vi "LIA-SR865A.vi"(0 "VISA resource name":refnum<visa-resource-name>="LIA", 1 "SubVI":bool, 5 "Input cluster":T1, 11 "error in (no error)":errorcluster) -> (4 "VISA resource name out":refnum<visa-resource-name>, 6 "output cluster":T1, 15 "error out":errorcluster)   [LabVIEW 2016]
uses:
  <instrlib>/Stanford Research SR865/Stanford Research SR865.lvlib
panel:
  out "On":bool
  out "On":bool
  in  "?":bool
  in  "?":bool
  out "On":bool
  out "On":bool
  in  "?":bool
  in  "?":bool
  in  "?":bool
  out "On":bool
  in  "?":bool
  out "On":bool
  in  "CH2 Offset":dbl min=-999.99 max=999.99 format="%#.2f"
  in  "CH1 Offset":dbl min=-999.99 max=999.99 format="%#.2f"
  in  "?":i32=1 min=1 max=99 step=1
  in  "?":bool
  out "On":bool
  in  "Trig":string(combo)="0"
  in  "?":bool
  out "On":bool
  in  "Slope":string(combo)="3"
  in  "Range":enum32{"1 mA", "10 nA"}(radio)
  in  "0":string(combo)="0"
  in  "Input":enum32{"50 W", "1 MW"}(radio)=enum."1 MW"
  in  "?":bool
  in  "Input Shields":enum32{"Float", "Ground"}(radio)=enum."Ground"
  in  "Couple":enum32{"AC", "DC"}(radio)
  in  "A-B":enum32{"A", "A-B"}(radio)
  in  "Mode":enum32{"Common", "Difference"}(radio)
  in  "Input":enum32{"Voltage", "Current"}(radio)
  in  "?":bool
  in  "DC Level":dbl min=-5.0 max=5.0 format="%.3f"
  in  "?":bool
  in  "Input Range":string(combo)="1"
  in  "?":bool
  in  "Amplitude":dbl=2.0 min=1e-09 max=2.0 format="%.3g"
  in  "Internal Ref\nFrequency":dbl=25.0 min=0.0 format="%.4f"
  in  "?":ext=-1.9354838709677438 format="%#.3g"
  in  "Expand":string(combo)="0"
  in  "CH2 Output":string(combo)="1"
  in  "Expand":string(combo)="0"
  in  "CH1 Output":string(combo)="1"
  in  "1":string(combo)="1"
  in  "Time Constant":string(combo)="0"
  in  "1":string(combo)="1"
  in  "Sensitivity":string(combo)="0"
  # "Signal"
  # "Reference"
  # "Sine Out"
  # "Phase"
  # "V"
  # "V"
  # "mV"
  # "External"
  # "Ref Source"
  # "kHz"
  # "Current"
  # "Voltage"
  # "Harmonic"
  # "Output"
  # "%"
  # "%"
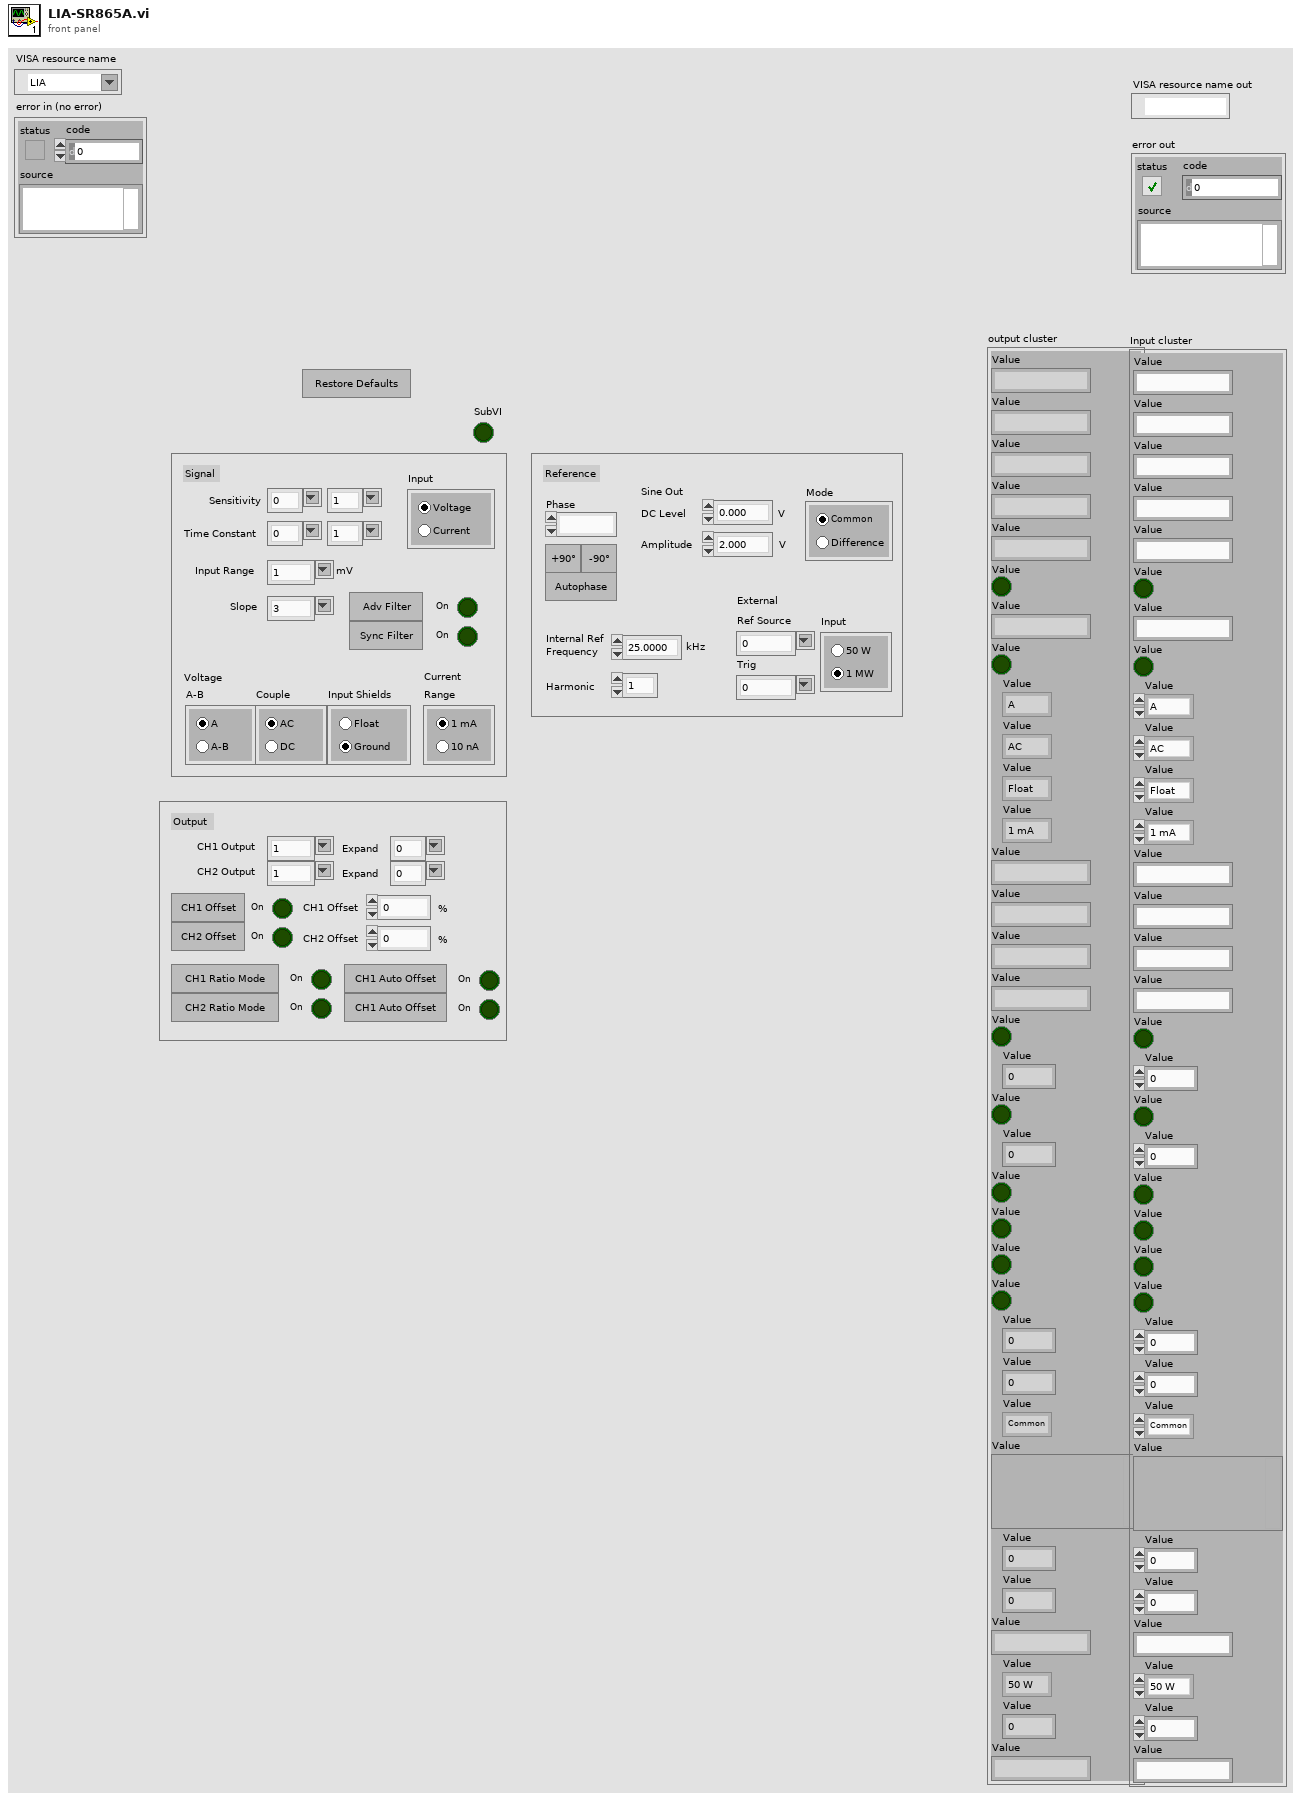
[diagram p1: front panel]
types:
  T1 = cluster{"Value":string, "Value":string, "Value":string, "Value":string, "Value":string, "Value":bool, "Value":string, "Value":bool, "Value":enum32{"A", "A-B"}, "Value":enum32{"AC", "DC"}, "Value":enum32{"Float", "Ground"}, "Value":enum32{"1 mA", "10 nA"}, "Value":string, "Value":string, "Value":string, "Value":string, "Value":bool, "Value":dbl, "Value":bool, "Value":dbl, "Value":bool, "Value":bool, "Value":bool, "Value":bool, "Value":ext, "Value":dbl, "Value":enum32{"Common", "Difference"}, "Value":variant, "Value":dbl, "Value":dbl, "Value":string, "Value":enum32{"50 W", "1 MW"}, "Value":i32, "Value":string}
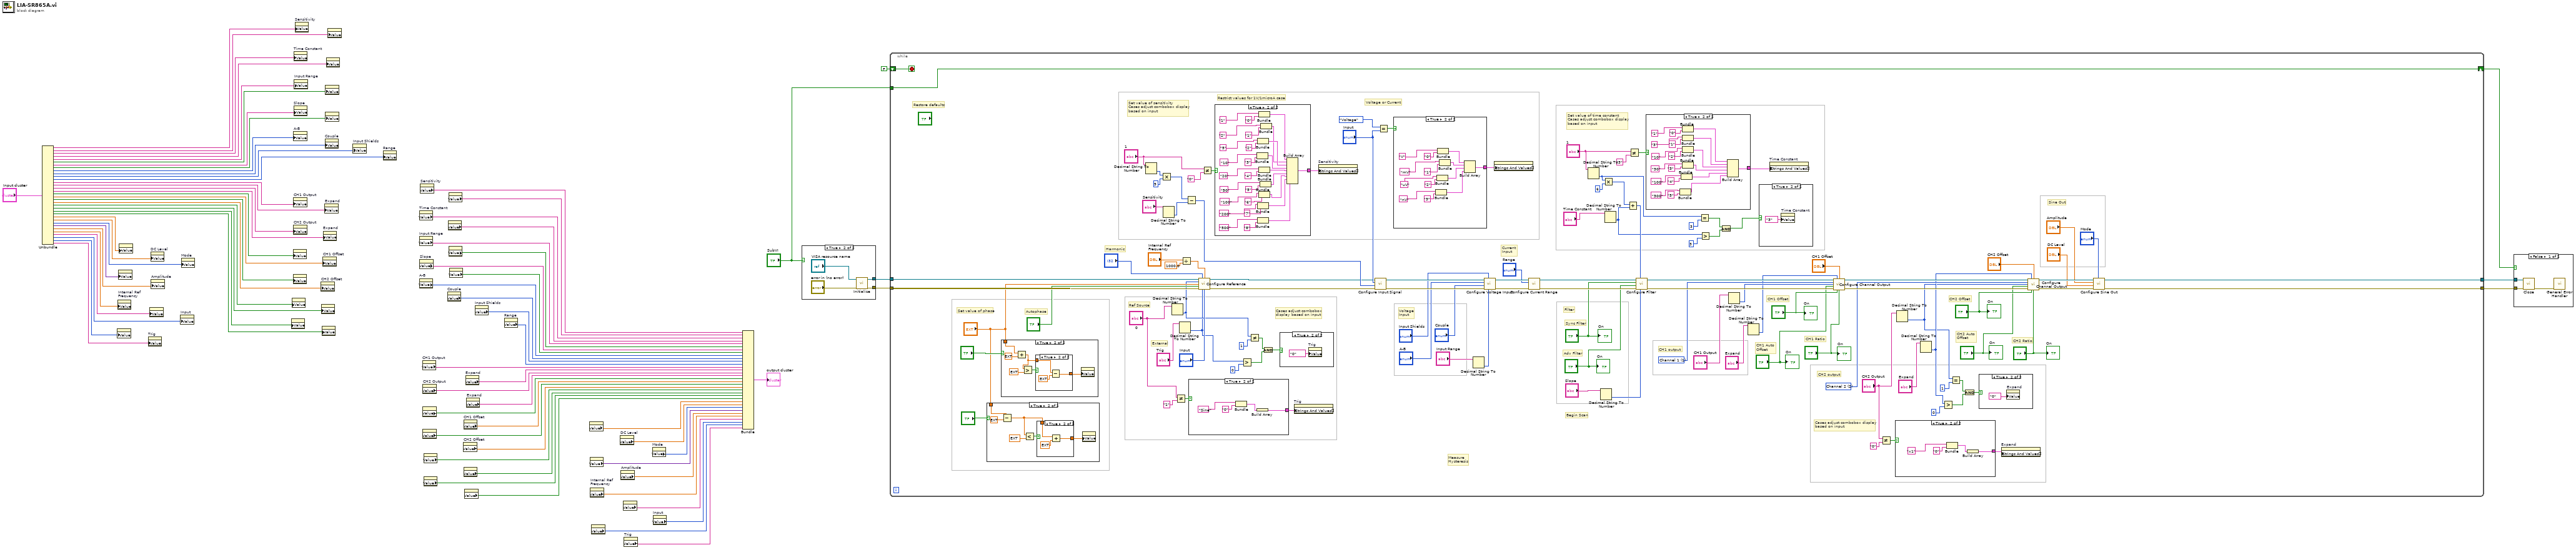
[diagram p0: block diagram]
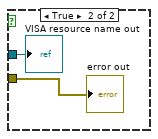
[diagram p2: hidden frame]
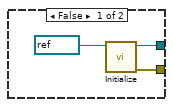
[diagram p3: hidden frame]
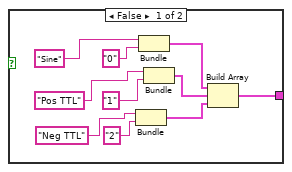
[diagram p4: hidden frame]
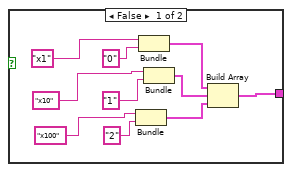
[diagram p7: hidden frame]
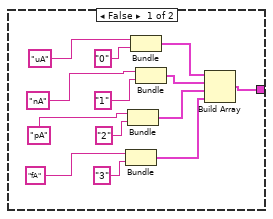
[diagram p9: hidden frame]
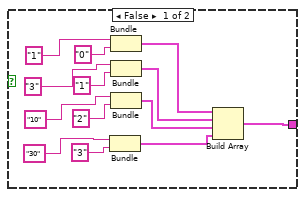
[diagram p14: hidden frame]
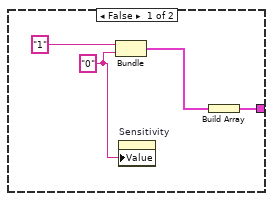
[diagram p15: hidden frame]
diagram:
  n1 = Unbundle("Input cluster") -> ("Value"=w42:string, "Value"=w41:string, "Value"=w40:string, "Value"=w39:string, "Value"=w38:string, "Value"=w37:bool, "Value"=w36:string, "Value"=w35:bool, "Value"=w34:enum32{"A", "A-B"}, "Value"=w33:enum32{"AC", "DC"}, "Value"=w32:enum32{"Float", "Ground"}, "Value"=w31:enum32{"1 mA", "10 nA"}, "Value"=w30:string, "Value"=w29:string, "Value"=w28:string, "Value"=w27:string, "Value"=w26:bool, "Value"=w25:dbl, "Value"=w24:bool, "Value"=w23:dbl, "Value"=w22:bool, "Value"=w21:bool, "Value"=w20:bool, "Value"=w19:bool, "Value"=w18:ext, "Value"=w17:dbl, "Value"=w16:enum32{"Common", "Difference"}, "Value"=w15:variant, "Value"=w14:dbl, "Value"=w13:dbl, "Value"=w12:string, "Value"=w11:enum32{"50 W", "1 MW"}, "Value"=w10:i32, "Value"=w9:string)
  n2 = property class="DigNum (strict)"("Value"=w10) -> ()  [unwired: 2 in, 2 out]
  n3 = property on="Internal Ref\nFrequency" class="DigNum (strict)"("Value"=w13) -> ()  [unwired: 2 in, 2 out]
  n4 = property class="Bool"("Value"=w15) -> ()  [unwired: 2 in, 2 out]
  n5 = property class="DigNum (strict)"("Value"=w18) -> ()  [unwired: 2 in, 2 out]
  n6 = property on="Trig" class="CmbBox"("Value"=w9) -> ()  [unwired: 2 in, 2 out]
  n7 = property class="CmbBox"("Value"=w12) -> ()  [unwired: 2 in, 2 out]
  n8 = property on="DC Level" class="DigNum (strict)"("Value"=w17) -> ()  [unwired: 2 in, 2 out]
  n9 = property on="Amplitude" class="DigNum (strict)"("Value"=w14) -> ()  [unwired: 2 in, 2 out]
  n10 = property on="Input" class="RadioBtnsControl (strict)"("Value"=w11) -> ()  [unwired: 2 in, 2 out]
  n11 = property on="Mode" class="RadioBtnsControl (strict)"("Value"=w16) -> ()  [unwired: 2 in, 2 out]
  n12 = property class="Bool (strict)"("Value"=w20) -> ()  [unwired: 2 in, 2 out]
  n13 = property class="Bool (strict)"("Value"=w22) -> ()  [unwired: 2 in, 2 out]
  n14 = property class="Bool (strict)"("Value"=w26) -> ()  [unwired: 2 in, 2 out]
  n15 = property class="Bool (strict)"("Value"=w24) -> ()  [unwired: 2 in, 2 out]
  n16 = property on="A-B" class="RadioBtnsControl (strict)"("Value"=w34) -> ()  [unwired: 2 in, 2 out]
  n17 = property on="CH1 Output" class="CmbBox"("Value"=w30) -> ()  [unwired: 2 in, 2 out]
  n18 = property on="CH2 Output" class="CmbBox"("Value"=w28) -> ()  [unwired: 2 in, 2 out]
  n19 = property on="Time Constant" class="CmbBox"("Value"=w40) -> ()  [unwired: 2 in, 2 out]
  n20 = property on="Slope" class="CmbBox"("Value"=w36) -> ()  [unwired: 2 in, 2 out]
  n21 = property on="Input Range" class="CmbBox"("Value"=w38) -> ()  [unwired: 2 in, 2 out]
  n22 = property on="Sensitivity" class="CmbBox"("Value"=w42) -> ()  [unwired: 2 in, 2 out]
  n23 = property on="CH2 Offset" class="DigNum (strict)"("Value"=w23) -> ()  [unwired: 2 in, 2 out]
  n24 = property class="Bool (strict)"("Value"=w21) -> ()  [unwired: 2 in, 2 out]
  n25 = property class="Bool (strict)"("Value"=w19) -> ()  [unwired: 2 in, 2 out]
  n26 = property on="CH1 Offset" class="DigNum (strict)"("Value"=w25) -> ()  [unwired: 2 in, 2 out]
  n27 = property on="Expand" class="CmbBox"("Value"=w27) -> ()  [unwired: 2 in, 2 out]
  n28 = property on="Expand" class="CmbBox"("Value"=w29) -> ()  [unwired: 2 in, 2 out]
  n29 = property on="Couple" class="RadioBtnsControl (strict)"("Value"=w33) -> ()  [unwired: 2 in, 2 out]
  n30 = property class="Bool (strict)"("Value"=w37) -> ()  [unwired: 2 in, 2 out]
  n31 = property class="Bool (strict)"("Value"=w35) -> ()  [unwired: 2 in, 2 out]
  n32 = property class="CmbBox"("Value"=w39) -> ()  [unwired: 2 in, 2 out]
  n33 = property class="CmbBox"("Value"=w41) -> ()  [unwired: 2 in, 2 out]
  n34 = property on="Input Shields" class="RadioBtnsControl (strict)"("Value"=w32) -> ()  [unwired: 2 in, 2 out]
  n35 = property on="Range" class="RadioBtnsControl (strict)"("Value"=w31) -> ()  [unwired: 2 in, 2 out]
  n36 = property on="Time Constant" class="CmbBox"() -> ("Value"=w74:string)  [unwired: 2 in, 2 out]
  n37 = property on="Input Range" class="CmbBox"() -> ("Value"=w72:string)  [unwired: 2 in, 2 out]
  n38 = property on="A-B" class="RadioBtnsControl (strict)"() -> ("Value"=w68:enum32{"A", "A-B"})  [unwired: 2 in, 2 out]
  n39 = property on="Slope" class="CmbBox"() -> ("Value"=w70:string)  [unwired: 2 in, 2 out]
  n40 = property on="Sensitivity" class="CmbBox"() -> ("Value"=w76:string)  [unwired: 2 in, 2 out]
  n41 = property on="CH1 Output" class="CmbBox"() -> ("Value"=w64:string)  [unwired: 2 in, 2 out]
  n42 = property on="CH2 Output" class="CmbBox"() -> ("Value"=w62:string)  [unwired: 2 in, 2 out]
  n43 = property class="Bool (strict)"() -> ("Value"=w60:bool)  [unwired: 2 in, 2 out]
  n44 = property class="Bool (strict)"() -> ("Value"=w58:bool)  [unwired: 2 in, 2 out]
  n45 = property class="Bool (strict)"() -> ("Value"=w56:bool)  [unwired: 2 in, 2 out]
  n46 = property class="Bool (strict)"() -> ("Value"=w54:bool)  [unwired: 2 in, 2 out]
  n47 = property on="Couple" class="RadioBtnsControl (strict)"() -> ("Value"=w67:enum32{"AC", "DC"})  [unwired: 2 in, 2 out]
  n48 = property class="CmbBox"() -> ("Value"=w73:string)  [unwired: 2 in, 2 out]
  n49 = property class="CmbBox"() -> ("Value"=w75:string)  [unwired: 2 in, 2 out]
  n50 = property class="Bool (strict)"() -> ("Value"=w71:bool)  [unwired: 2 in, 2 out]
  n51 = property class="Bool (strict)"() -> ("Value"=w69:bool)  [unwired: 2 in, 2 out]
  n52 = property on="CH2 Offset" class="DigNum (strict)"() -> ("Value"=w57:dbl)  [unwired: 2 in, 2 out]
  n53 = property on="CH1 Offset" class="DigNum (strict)"() -> ("Value"=w59:dbl)  [unwired: 2 in, 2 out]
  n54 = property class="Bool (strict)"() -> ("Value"=w55:bool)  [unwired: 2 in, 2 out]
  n55 = property class="Bool (strict)"() -> ("Value"=w53:bool)  [unwired: 2 in, 2 out]
  n56 = property on="Expand" class="CmbBox"() -> ("Value"=w63:string)  [unwired: 2 in, 2 out]
  n57 = property on="Expand" class="CmbBox"() -> ("Value"=w61:string)  [unwired: 2 in, 2 out]
  n58 = property on="Input Shields" class="RadioBtnsControl (strict)"() -> ("Value"=w66:enum32{"Float", "Ground"})  [unwired: 2 in, 2 out]
  n59 = property on="Range" class="RadioBtnsControl (strict)"() -> ("Value"=w65:enum32{"1 mA", "10 nA"})  [unwired: 2 in, 2 out]
  n60 = property class="DigNum (strict)"() -> ("Value"=w52:ext)  [unwired: 2 in, 2 out]
  n61 = property class="Bool"() -> ("Value"=w49:variant)  [unwired: 2 in, 2 out]
  n62 = property on="Internal Ref\nFrequency" class="DigNum (strict)"() -> ("Value"=w47:dbl)  [unwired: 2 in, 2 out]
  n63 = property class="DigNum (strict)"() -> ("Value"=w44:i32)  [unwired: 2 in, 2 out]
  n64 = property on="DC Level" class="DigNum (strict)"() -> ("Value"=w51:dbl)  [unwired: 2 in, 2 out]
  n65 = property on="Amplitude" class="DigNum (strict)"() -> ("Value"=w48:dbl)  [unwired: 2 in, 2 out]
  n66 = property class="CmbBox"() -> ("Value"=w46:string)  [unwired: 2 in, 2 out]
  n67 = property on="Trig" class="CmbBox"() -> ("Value"=w43:string)  [unwired: 2 in, 2 out]
  n68 = property on="Mode" class="RadioBtnsControl (strict)"() -> ("Value"=w50:enum32{"Common", "Difference"})  [unwired: 2 in, 2 out]
  n69 = property on="Input" class="RadioBtnsControl (strict)"() -> ("Value"=w45:enum32{"50 W", "1 MW"})  [unwired: 2 in, 2 out]
  n70 = Bundle("Value"=w76, "Value"=w75, "Value"=w74, "Value"=w73, "Value"=w72, "Value"=w71, "Value"=w70, "Value"=w69, "Value"=w68, "Value"=w67, "Value"=w66, "Value"=w65, "Value"=w64, "Value"=w63, "Value"=w62, "Value"=w61, "Value"=w60, "Value"=w59, "Value"=w58, "Value"=w57, "Value"=w56, "Value"=w55, "Value"=w54, "Value"=w53, "Value"=w52, "Value"=w51, "Value"=w50, "Value"=w49, "Value"=w48, "Value"=w47, "Value"=w46, "Value"=w45, "Value"=w44, "Value"=w43) -> (→"output cluster":T1)  [unwired: 1 in]
  n71 = case shown="True" "SubVI" {
    tunnel: [w79 w84] -> w6
    tunnel: [w78 w83] -> w5
    frame False {
      n72 = call <instrlib>:"Initialize.vi"("VISA resource name"=refnum<visa-resource-name> "LIA") -> ("error out"=w78:errorcluster, "VISA resource name out"=w79:refnum<visa-resource-name>)  [unwired: 9 in]
    }
    frame True {
      n73 = call <instrlib>:"Initialize.vi"("error in (no error)"="error in (no error)", "VISA resource name"="VISA resource name") -> ("error out"=w83:errorcluster, "VISA resource name out"=w84:refnum<visa-resource-name>)  [unwired: 8 in]
    }
  }
  n74 = while {
    tunnel: w6 -> [w180]
    tunnel: w5 -> [w179]
    tunnel: [w87] -> w4
    tunnel: [w86] -> w3
    shift-right: [w85] -> w2
    shift-left: FALSE ("SubVI") -> [w93]
    tunnel: "SubVI" -> [w85]
    stop <- w93 stop-if-true
    w132 = 2 items=["Channel 1"=1, "Channel 2"=2] ("Channel Name (1: Channel 1)")
    w133 = 1 items=["Channel 1"=1, "Channel 2"=2] ("Channel Name (1: Channel 1)")
    # "CH2 Auto\nOffset"
    # "CH1 Auto\nOffset"
    # "CH1 Ratio"
    # "CH2 Ratio"
    # "CH2 Offset"
    # "CH1 Offset"
    # "Sine Out"
    # "Cases adjust combobox\ndisplay based on input"
    # "Cases adjust combobox display\nbased on input"
    # "CH2 output"
    # "Filter"
    # "Current\nInput"
    # "Sync Filter"
    # "Restrict values for 1V/1microA case"
    # "Voltage or Current"
    # "Autophase"
    # "Harmonic"
    # "Begin Scan"
    # "Measure\nHysteresis"
    # "Ref Source"
    # "External"
    # "Adv Filter"
    # "Restore defaults"
    # "Voltage\nInput"
    # "Set value of phase"
    # "CH1 output"
    # "Set value of time constant\nCases adjust combobox display\nbased on input"
    # "Set value of sensitivity\nCases adjust combobox display\nbased on input"
    n75 = case shown="True" "?" {
      tunnel: "?" -> [_ w266]
      frame False {
      }
      frame True {
        n76 = Subtract(x=w266, y=ext 90.0) -> (x-y=w262:ext)
        n77 = Less?(x=w262, y=ext -180.0) -> (x < y?=w263:bool)
        n78 = case shown="True" w263 {
          tunnel: w262 -> [w267 w269]
          tunnel: [w267 w268] -> w261
          frame False {
          }
          frame True {
            n79 = Add(x=w269, y=ext 360.0) -> (x+y=w268:ext)
          }
        }
        n80 = property class="DigNum (strict)"("Value"=w261) -> ()  [unwired: 2 in, 2 out]
      }
    }
    n81 = case shown="True" "?" {
      tunnel: "?" -> [_ w256]
      frame False {
      }
      frame True {
        n82 = Add(x=w256, y=ext 90.0) -> (x+y=w252:ext)
        n83 = Greater?(x=w252, y=ext 180.0) -> (0:w254:bool)
        n84 = case shown="True" w254 {
          tunnel: w252 -> [w257 w260]
          tunnel: [w257 w258] -> w251
          frame False {
          }
          frame True {
            n85 = Subtract(x=w260, y=ext 360.0) -> (x-y=w258:ext)
          }
        }
        n86 = property class="DigNum (strict)"("Value"=w251) -> ()  [unwired: 2 in, 2 out]
      }
    }
    n87 = Decimal String To Number(string="1") -> (number=w176:i32)  [unwired: 2 in, 1 out]
    n88 = Multiply(x=w176, y=9) -> (x*y=w173:i32)
    n89 = Decimal String To Number(string="Sensitivity") -> (number=w174:i32)  [unwired: 2 in, 1 out]
    n90 = Decimal String To Number(string="0") -> (number=w114:i32)  [unwired: 2 in, 1 out]
    n91 = Not Equal?(x="0", y="1") -> (x != y?=w109:bool)
    n92 = Decimal String To Number(string="Trig") -> (number=w112:i32)  [unwired: 2 in, 1 out]
    n93 = Divide(x="Internal Ref\nFrequency", y=1000.0) -> (x/y=w89:dbl)
    n94 = Subtract(x=w173, y=w174) -> (x-y=w149:i32)
    n95 = case shown="True" w109 {
      tunnel: [w197 w204] -> w108
      frame False {
        n96 = Bundle("Neg TTL", "2") -> (w194:cluster{string, string})  [unwired: 1 in]
        n97 = Bundle("Sine", "0") -> (w196:cluster{string, string})  [unwired: 1 in]
        n98 = Bundle("Pos TTL", "1") -> (w195:cluster{string, string})  [unwired: 1 in]
        n99 = Build Array(w196, w195, w194) -> (w197:cluster{string, string}[])
      }
      frame True {
        n100 = Bundle("Sine", "0") -> (w205:cluster{string, string})  [unwired: 1 in]
        n101 = Build Array(w205) -> (w204:cluster{string, string}[])
      }
    }
    n102 = call <instrlib>:"Configure Reference.vi"("VISA resource name"=w180, "Detection Harmonic Number (1)"="?", "Internal Reference Frequency (100000Hz)"=w89, "Reference Source (0: Internal)"=w114, "Manual Phase (0 Degree)"="?", "Auto Phase(0:Disabled)"="?", "error in (no error)"=w179, "External Reference Trigger (0: Sine Zero Crossing)"=w112, "External Reference Trigger Input (0: 50OHMS)"="Input") -> ("VISA resource name out"=w92:refnum<visa-resource-name>, "error out"=w91:errorcluster)  [unwired: 5 in]
    n103 = Not Equal?(x="1", y="0") -> (x != y?=w193:bool)
    n104 = case shown="True" w193 {
      tunnel: [w305 w307] -> w172
      frame False {
        w303 = "0"
        n105 = Bundle("1", w303) -> (w304:cluster{string, string})  [unwired: 1 in]
        n106 = property on="Sensitivity" class="CmbBox"("Value"=w303) -> ()  [unwired: 2 in, 2 out]
        n107 = Build Array(w304) -> (w305:cluster{string, string}[])
      }
      frame True {
        n108 = Bundle("10", "3") -> (w331:cluster{string, string})  [unwired: 1 in]
        n109 = Bundle("5", "2") -> (w333:cluster{string, string})  [unwired: 1 in]
        n110 = Bundle("200", "7") -> (w327:cluster{string, string})  [unwired: 1 in]
        n111 = Bundle("500", "8") -> (w326:cluster{string, string})  [unwired: 1 in]
        n112 = Bundle("1", "0") -> (w334:cluster{string, string})  [unwired: 1 in]
        n113 = Bundle("100", "6") -> (w328:cluster{string, string})  [unwired: 1 in]
        n114 = Bundle("20", "4") -> (w330:cluster{string, string})  [unwired: 1 in]
        n115 = Bundle("50", "5") -> (w329:cluster{string, string})  [unwired: 1 in]
        n116 = Bundle("2", "1") -> (w332:cluster{string, string})  [unwired: 1 in]
        n117 = Build Array(w334, w332, w333, w331, w330, w329, w328, w327, w326) -> (w307:cluster{string, string}[])
      }
    }
    n118 = Greater?(x=w112, y=0) -> (0:w115:bool)
    n119 = Not Equal?(x=w114, y=1) -> (x != y?=w113:bool)
    n120 = And(x=w113, y=w115) -> (x .and. y?=w111:bool)
    n121 = case shown="True" w111 {
      frame False {
      }
      frame True {
        n122 = property on="Trig" class="CmbBox"("Value"="0" ("Trig")) -> ()  [unwired: 2 in, 2 out]
      }
    }
    n123 = property on="Trig" class="CmbBox"("Strings And Values[]"=w108) -> ()  [unwired: 2 in, 2 out]
    n124 = property on="Sensitivity" class="CmbBox"("Strings And Values[]"=w172) -> ()  [unwired: 2 in, 2 out]
    n125 = call <instrlib>:"Configure Input Signal.vi"("error in (no error)"=w91, "Sensitivity (0: 1 V [uA])"=w149, "Signal Input (0: Voltage)"="Input", "VISA resource name"=w92) -> ("error out"=w185:errorcluster, "VISA resource name out"=w181:refnum<visa-resource-name>)  [unwired: 6 in]
    n126 = Equal?(x=enum32{"Voltage", "Current"}."Voltage" ("y"), y="Input") -> (x = y?=w168:bool)
    n127 = case shown="True" w168 {
      tunnel: [w225 w242] -> w167
      frame False {
        n128 = Bundle("fA", "3") -> (w226:cluster{string, string})  [unwired: 1 in]
        n129 = Bundle("pA", "2") -> (w227:cluster{string, string})  [unwired: 1 in]
        n130 = Bundle("uA", "0") -> (w229:cluster{string, string})  [unwired: 1 in]
        n131 = Bundle("nA", "1") -> (w228:cluster{string, string})  [unwired: 1 in]
        n132 = Build Array(w229, w228, w227, w226) -> (w225:cluster{string, string}[])
      }
      frame True {
        n133 = Bundle("nV", "3") -> (w238:cluster{string, string})  [unwired: 1 in]
        n134 = Bundle("uV", "2") -> (w239:cluster{string, string})  [unwired: 1 in]
        n135 = Bundle("V", "0") -> (w241:cluster{string, string})  [unwired: 1 in]
        n136 = Bundle("mV", "1") -> (w240:cluster{string, string})  [unwired: 1 in]
        n137 = Build Array(w241, w240, w239, w238) -> (w242:cluster{string, string}[])
      }
    }
    n138 = Decimal String To Number(string="Input Range") -> (number=w140:i32)  [unwired: 2 in, 1 out]
    n139 = call <instrlib>:"Configure Voltage Input.vi"("Voltage Input Range (0: 1V)"=w140, "Voltage Input Shields (0: Float)"="Input Shields", "error in (no error)"=w185, "Voltage Input Coupling (0: AC)"="Couple", "Voltage Input Mode (0: A)"="A-B", "VISA resource name"=w181) -> ("error out"=w186:errorcluster, "VISA resource name out"=w182:refnum<visa-resource-name>)  [unwired: 4 in]
    n140 = property class="CmbBox"("Strings And Values[]"=w167) -> ()  [unwired: 2 in, 2 out]
    n141 = call <instrlib>:"Configure Current Range.vi"("error in (no error)"=w186, "Current Input Gain (0: 1MOmega(1uA))"="Range", "VISA resource name"=w182) -> ("error out"=w187:errorcluster, "VISA resource name out"=w183:refnum<visa-resource-name>)  [unwired: 7 in]
    n142 = Decimal String To Number(string="1") -> (number=w161:i32)  [unwired: 2 in, 1 out]
    n143 = Decimal String To Number(string="Slope") -> (number=w152:i32)  [unwired: 2 in, 1 out]
    n144 = Multiply(x=w161, y=6) -> (x*y=w165:i32)
    n145 = Decimal String To Number(string="Time Constant") -> (number=w160:i32)  [unwired: 2 in, 1 out]
    n146 = Add(x=w165, y=w160) -> (x+y=w162:i32)
    n147 = Not Equal?(x="1", y="3") -> (x != y?=w191:bool)
    n148 = call <instrlib>:"Configure Filter.vi"("Filter Slope (0: 6 dB/oct)"=w152, "Time Constant (10: 100 ms)"=w162, "error in (no error)"=w187, "Advanced Filter (0: OFF)"="?", "Sync Filter (0: OFF)"="?", "VISA resource name"=w183) -> ("error out"=w188:errorcluster, "VISA resource name out"=w184:refnum<visa-resource-name>)  [unwired: 4 in]
    n149 = case shown="True" w191 {
      tunnel: [w276 w284] -> w155
      frame False {
        n150 = Bundle("30", "3") -> (w272:cluster{string, string})  [unwired: 1 in]
        n151 = Bundle("1", "0") -> (w275:cluster{string, string})  [unwired: 1 in]
        n152 = Bundle("3", "1") -> (w274:cluster{string, string})  [unwired: 1 in]
        n153 = Bundle("10", "2") -> (w273:cluster{string, string})  [unwired: 1 in]
        n154 = Build Array(w275, w274, w273, w272) -> (w276:cluster{string, string}[])
      }
      frame True {
        n155 = Bundle("300", "5") -> (w285:cluster{string, string})  [unwired: 1 in]
        n156 = Bundle("100", "4") -> (w286:cluster{string, string})  [unwired: 1 in]
        n157 = Bundle("30", "3") -> (w287:cluster{string, string})  [unwired: 1 in]
        n158 = Bundle("1", "0") -> (w290:cluster{string, string})  [unwired: 1 in]
        n159 = Bundle("3", "1") -> (w289:cluster{string, string})  [unwired: 1 in]
        n160 = Bundle("10", "2") -> (w288:cluster{string, string})  [unwired: 1 in]
        n161 = Build Array(w290, w289, w288, w287, w286, w285) -> (w284:cluster{string, string}[])
      }
    }
    n162 = Equal?(x=w161, y=3) -> (x = y?=w156:bool)
    n163 = Greater?(x=w160, y=3) -> (0:w157:bool)
    n164 = And(x=w156, y=w157) -> (x .and. y?=w154:bool)
    n165 = Decimal String To Number(string="CH1 Output") -> (number=w134:i32)  [unwired: 2 in, 1 out]
    n166 = Decimal String To Number(string="Expand") -> (number=w130:i32)  [unwired: 2 in, 1 out]
    n167 = case shown="True" w154 {
      frame False {
      }
      frame True {
        n168 = property on="Time Constant" class="CmbBox"("Value"="3" ("Time Constant")) -> ()  [unwired: 2 in, 2 out]
      }
    }
    n169 = property on="Time Constant" class="CmbBox"("Strings And Values[]"=w155) -> ()  [unwired: 2 in, 2 out]
    n170 = call <instrlib>:"Configure Channel Output.vi"("VISA resource name"=w184, "Output Expand Mode (0: OFF)"=w130, "Output Offset Percentage (0)"="CH1 Offset", "Channel Name (1: Channel 1)"=w133, "Channel Output (0: XY)"=w134, "Auto Offset State (0: OFF)"="?", "error in (no error)"=w188, "Output Offset State (0: OFF)"="?", "Ratio Mode (0: OFF)"="?") -> ("VISA resource name out"=w137:refnum<visa-resource-name>, "error out"=w136:errorcluster)  [unwired: 5 in]
    n171 = Not Equal?(x="CH2 Output", y="0") -> (x != y?=w126:bool)
    n172 = case shown="True" w126 {
      tunnel: [w213 w220] -> w125
      frame False {
        n173 = Bundle("x100", "2") -> (w210:cluster{string, string})  [unwired: 1 in]
        n174 = Bundle("x1", "0") -> (w212:cluster{string, string})  [unwired: 1 in]
        n175 = Bundle("x10", "1") -> (w211:cluster{string, string})  [unwired: 1 in]
        n176 = Build Array(w212, w211, w210) -> (w213:cluster{string, string}[])
      }
      frame True {
        n177 = Bundle("x1", "0") -> (w221:cluster{string, string})  [unwired: 1 in]
        n178 = Build Array(w221) -> (w220:cluster{string, string}[])
      }
    }
    n179 = Decimal String To Number(string="CH2 Output") -> (number=w119:i32)  [unwired: 2 in, 1 out]
    n180 = Decimal String To Number(string="Expand") -> (number=w123:i32)  [unwired: 2 in, 1 out]
    n181 = Greater?(x=w123, y=0) -> (0:w121:bool)
    n182 = Equal?(x=w119, y=1) -> (x = y?=w120:bool)
    n183 = And(x=w120, y=w121) -> (x .and. y?=w118:bool)
    n184 = case shown="True" w118 {
      frame False {
      }
      frame True {
        n185 = property on="Expand" class="CmbBox"("Value"="0" ("Expand")) -> ()  [unwired: 2 in, 2 out]
      }
    }
    n186 = property on="Expand" class="CmbBox"("Strings And Values[]"=w125) -> ()  [unwired: 2 in, 2 out]
    n187 = call <instrlib>:"Configure Channel Output.vi"("VISA resource name"=w137, "Output Expand Mode (0: OFF)"=w123, "Output Offset Percentage (0)"="CH2 Offset", "Channel Name (1: Channel 1)"=w132, "Channel Output (0: XY)"=w119, "Auto Offset State (0: OFF)"="?", "error in (no error)"=w136, "Output Offset State (0: OFF)"="?", "Ratio Mode (0: OFF)"="?") -> ("VISA resource name out"=w106:refnum<visa-resource-name>, "error out"=w105:errorcluster)  [unwired: 5 in]
    n188 = call <instrlib>:"Configure Sine Out.vi"("Sine Out DC Level Mode (0: Common)"="Mode", "error in (no error)"=w105, "Sine Out DC Level to Voltage (0 V)"="DC Level", "Sine Out Amplitude to Voltage (0 V)"="Amplitude", "VISA resource name"=w106) -> ("error out"=w86:errorcluster, "VISA resource name out"=w87:refnum<visa-resource-name>)  [unwired: 5 in]
    "On" <- "?"
    "On" <- "?"
    "On" <- "?"
    "On" <- "?"
    "On" <- "?"
    "On" <- "?"
    "On" <- "?"
    "On" <- "?"
  }
  n189 = case shown="False" w2 {
    tunnel: w3 -> [w335 w338]
    tunnel: w4 -> [w336 w339]
    frame False {
      n190 = call <instrlib>:"Close.vi"("error in (no error)"=w335, "VISA resource name"=w336) -> ("error out"=w337:errorcluster)  [unwired: 9 in]
      n191 = call <vilib>:"General Error Handler.vi"("error in (no error)"=w337) -> ()  [unwired: 10 in, 5 out]
    }
    frame True {
      "VISA resource name out" <- w339
      "error out" <- w338
    }
  }
